vi "Enable Disable Controls.vi"(8 "error in (no error)":errorcluster, 10 "State Array":T1(array[ring]), 11 "Data Cluster":T2) -> (0 "error out":errorcluster)   [LabVIEW 2018]
doc: "Sets the enable/disable state for Connect, Disconnect, Subscribe, Unsubscribe and Publish buttons. Provide an array of enums in that order."
uses:
  controls/UI Data.ctl
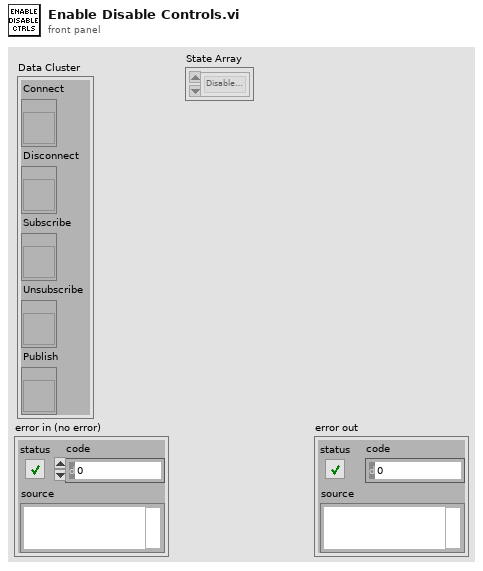
[diagram p1: front panel]
types:
  T1 = enum8{"Enabled", "Disabled", "Disabled and Grayed Out"}[]
  T2 = typedef "UI Data.ctl" = cluster{"Connect":refnum<vi>, "Disconnect":refnum<vi>, "Subscribe":refnum<vi>, "Unsubscribe":refnum<vi>, "Publish":refnum<vi>}
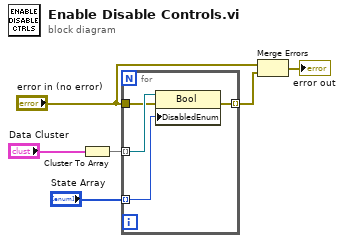
[diagram p0: block diagram]
diagram:
  n1 = Cluster To Array(cluster="Data Cluster") -> (array=w5:refnum<vi>[])
  n2 = for {
    tunnel: w5 -> [w10] mode=indexing
    tunnel: "State Array" -> [w9] mode=indexing
    tunnel: [w8] -> w3 mode=indexing
    tunnel: "error in (no error)" -> [w7]
    n3 = property class="Bool"(reference=w10, error in=w7, "DisabledEnum"=w9) -> (error out=w8:errorcluster)  [unwired: 1 out]
  }
  n4 = Merge Errors("error in (no error)", w3) -> (→"error out":errorcluster)
